vi "Update Version.vi"(8 "error in (no error)":errorcluster, 11 "NamedPackage in":refnum<class "NamedPackage.lvclass">) -> (0 "error out":errorcluster, 3 "NamedPackage out":refnum<class "NamedPackage.lvclass">)   [LabVIEW 2020, in "GPack.lvlib" / "NamedPackage.lvclass"]
uses:
  NamedPackage.lvclass
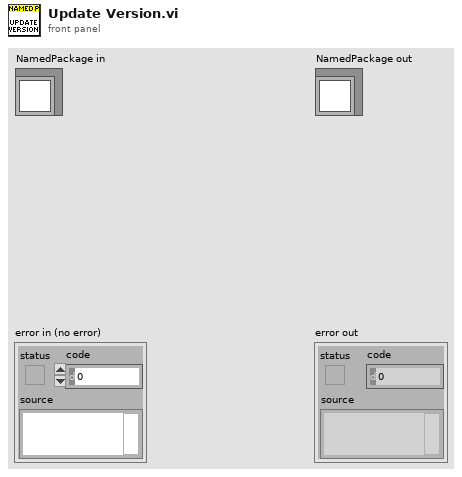
[diagram p1: front panel]
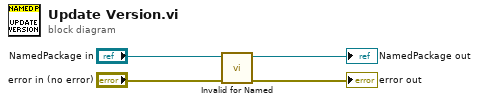
[diagram p0: block diagram]
diagram:
  n1 = call "Invalid for Named.vi"("error in (no error)"="error in (no error)", "NamedPackage in"="NamedPackage in") -> ("error out"=→"error out":errorcluster, "NamedPackage out"=→"NamedPackage out":refnum<class "NamedPackage.lvclass">)  [unwired: 8 in]
